vi "Add Authentication.vi"   [LabVIEW 2020, in "wamplv.lvlib" / "WAMP Client.lvclass"]
uses:
  WAMP Client.lvclass
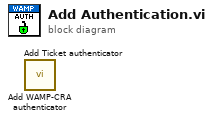
[diagram p0: block diagram]
diagram:
  n1 = call "Add WAMP-CRA authenticator.vi"() -> ()  [unwired: 10 in, 2 out]
  n2 = call "Add Ticket authenticator.vi"() -> ()  [unwired: 10 in, 2 out]
